vi "Rio_X_Motor_PID_Position_Control.vi"() -> ()   [LabVIEW 2017]
uses:
  <vilib>/myRIO/Common/Instrument Driver Framework/myRIO v1.0/Encoder/typedefs/Encoder Signal Mode.ctl
  <vilib>/myRIO/Instrument Drivers/Onboard IO/Encoder/typedefs/Encoder Reference.ctl
  <vilib>/myRIO/Common/Instrument Driver Framework/Utilities/typedefs/myRIO Generic Hardware Reference.ctl
  <vilib>/myRIO/Common/Instrument Driver Framework/Utilities/typedefs/Hardware Version Enum.ctl
  <vilib>/myRIO/Common/Instrument Driver Framework/Utilities/typedefs/myRIO v1.0 Reference.ctl
  <vilib>/myRIO/Common/Instrument Driver Framework/Utilities/typedefs/Generic FPGA Reference.ctl
  <vilib>/myRIO/Common/Instrument Driver Framework/myRIO v1.0/Encoder/typedefs/Encoder Channels Enum.ctl
  <vilib>/myRIO/Common/Instrument Driver Framework/myRIO v1.0/Encoder/typedefs/Encoder Configuration v1.0.ctl
  <vilib>/userdefined/High Color/nirio_resource_hc.ctl
  <vilib>/myRIO/Instrument Drivers/Onboard IO/DIO/typedefs/DIO Reference.ctl
  <vilib>/myRIO/Common/Instrument Driver Framework/myRIO v1.0/DIO/typedefs/DIO Channels List.ctl
  <vilib>/myRIO/Common/Instrument Driver Framework/myRIO v1.0/DIO/typedefs/DIO Channels Enum.ctl
  <vilib>/myRIO/Instrument Drivers/Onboard IO/PWM/typedefs/PWM Reference.ctl
  <vilib>/myRIO/Common/Instrument Driver Framework/myRIO v1.0/PWM/typedefs/PWM Channels Enum.ctl
  <vilib>/myRIO/Instrument Drivers/Onboard IO/PWM/typedefs/PWM Configuration.ctl
  <vilib>/myRIO/Common/Instrument Driver Framework/Utilities/vis/Is FPGA Ref Available.vi
  <vilib>/myRIO/Common/Instrument Driver Framework/myRIO v1.0/Encoder/vis/myRIO v1.1 Open Encoder.vi
  <vilib>/myRIO/Instrument Drivers/Onboard IO/Encoder/vis/Read.vi
  <vilib>/myRIO/Common/Instrument Driver Framework/myRIO v1.0/DIO/vis/myRIO v1.1 Open DIO.vi
  <vilib>/myRIO/Instrument Drivers/Onboard IO/DIO/vis/Write.vi
  <vilib>/myRIO/Common/Instrument Driver Framework/myRIO v1.0/PWM/vis/myRIO v1.1 Open PWM.vi
  <vilib>/myRIO/Instrument Drivers/Onboard IO/PWM/vis/Set Duty Cycle and Frequency.vi
  <vilib>/myRIO/Common/Instrument Driver Framework/Utilities/vis/Validate Channels.vi
  <vilib>/myRIO/Common/Instrument Driver Framework/myRIO v1.0/Encoder/vis/myRIO v1.0 Reserve Encoder.vi
  <vilib>/myRIO/Common/Instrument Driver Framework/myRIO v1.0/DIO/vis/myRIO v1.0 Reserve DIO.vi
  <vilib>/myRIO/Common/Instrument Driver Framework/myRIO v1.0/PWM/vis/myRIO v1.0 Reserve PWM.vi
  <vilib>/myRIO/Common/Instrument Driver Framework/myRIO v1.0/Encoder/vis/myRIO v1.0 Build MUX Configuration Encoder.vi
  <vilib>/myRIO/Common/Instrument Driver Framework/myRIO v1.0/Resource Manager/vis/myRIO v1.0 Reserve Channel List.vi
  <vilib>/myRIO/Common/Instrument Driver Framework/myRIO v1.0/DIO/vis/myRIO v1.0 Build MUX Configuration DIO.vi
  <vilib>/myRIO/Common/Instrument Driver Framework/myRIO v1.0/PWM/vis/myRIO v1.0 Build MUX Configuration PWM.vi
  <vilib>/myRIO/Common/Instrument Driver Framework/myRIO v1.0/Resource Manager/vis/myRIO v1.0 Create Configuration List.vi
  <vilib>/myRIO/Common/Instrument Driver Framework/myRIO v1.0/Resource Manager/vis/myRIO v1.0 Reserve Channel.vi
  <vilib>/myRIO/Common/Instrument Driver Framework/myRIO v1.0/Resource Manager/vis/myRIO v1.0 Unreserve Channel.vi
  <vilib>/myRIO/Common/Instrument Driver Framework/myRIO v1.0/Resource Manager/vis/myRIO v1.0 Build Mutex Name.vi
  <vilib>/Utility/VariantDataType/GetNumericInfo.vi
  <vilib>/Utility/error.llb/Error Cluster From Error Code.vi
  <vilib>/myRIO/Common/Instrument Driver Framework/myRIO v1.0/myRIO v1.1 Open.vi
  <vilib>/myRIO/Common/Instrument Driver Framework/Utilities/vis/IO Manager.vi
  <vilib>/myRIO/Common/Instrument Driver Framework/Utilities/vis/Configuration Manager.vi
  <vilib>/myRIO/Common/Instrument Driver Framework/myRIO v1.0/Resource Manager/vis/myRIO v1.0 Configure IO.vi
  <vilib>/myRIO/Common/Instrument Driver Framework/myRIO v1.0/myRIO v1.0 Close.vi
  <vilib>/myRIO/Common/Instrument Driver Framework/myRIO v1.0/Encoder/vis/myRIO v1.0 Configure Encoder.vi
  <vilib>/myRIO/Common/Instrument Driver Framework/myRIO v1.0/Encoder/vis/myRIO v1.0 Read Encoder.vi
  <vilib>/addons/control/pid/pid.llb/PID (DBL).vi
  <vilib>/myRIO/Common/Instrument Driver Framework/myRIO v1.0/DIO/vis/myRIO v1.0 Write DIO.vi
  <vilib>/myRIO/Common/Instrument Driver Framework/myRIO v1.0/PWM/vis/myRIO v1.0 Write PWM.vi
  <vilib>/myRIO/Express VI/Onboard IO/Encoder/Encoder Express VI.xnode
  <vilib>/myRIO/Instrument Drivers/Onboard IO/Encoder/vis/myRIO Encoder Open.xnode
  <vilib>/myRIO/Common/Instrument Driver Framework/myRIO v1.0/Encoder/typedefs/Encoder Count Direction Enum.ctl
  <vilib>/myRIO/Express VI/Onboard IO/DO/DO Express VI.xnode
  <vilib>/myRIO/Instrument Drivers/Onboard IO/DIO/vis/myRIO DIO Open.xnode
  <vilib>/myRIO/Express VI/Onboard IO/PWM/PWM Express VI.xnode
  <vilib>/myRIO/Instrument Drivers/Onboard IO/PWM/vis/myRIO PWM Open.xnode
  <vilib>/myRIO/Instrument Drivers/Onboard IO/Encoder/Encoder.lvlib
  <vilib>/addons/control/pid/NI_PID_pid.lvlib
  <vilib>/myRIO/Instrument Drivers/Onboard IO/PWM/PWM.lvlib
  <vilib>/myRIO/Instrument Drivers/Onboard IO/DIO/DIO.lvlib
  <vilib>/addons/control/pid/pid.llb/PID Control Input Filter (DBL).vi
panel:
  out "Waveform Chart":dbl[][](graph)
  in  "PID gains":T1={"proportional gain (Kc)"=1.0, "integral time (Ti, min)"=0.01, "derivative time (Td, min)"=0.0} {"derivative time (Td, min)" format="%.3f"; "integral time (Ti, min)" format="%.3f"; "proportional gain (Kc)" format="%.3f"}
  in  "setpoint":dbl format="%.2f"
  out "Counter Value 2":i32
  in  "stop 3":bool
  in  "stop 2":bool
  out "Error Out":errorcluster
  in  "Error In":errorcluster
  out "Waveform Graph":dbl[](graph)
  out "RPM Chart 2":cluster{"setpoint":dbl, dbl, "output":dbl}(graph)
  in  "Boolean":bool
  out "Time":dbl
  out "element":dbl
  in  "Controls":T2={"Start Pos"=0.0, "End Pos"=0.0, "Max V R/m"=100, "Accel Time (S)"=0.0}
  in  "stop":bool
  out "RPM Chart":dbl(graph)
  out "Counter Value":i32
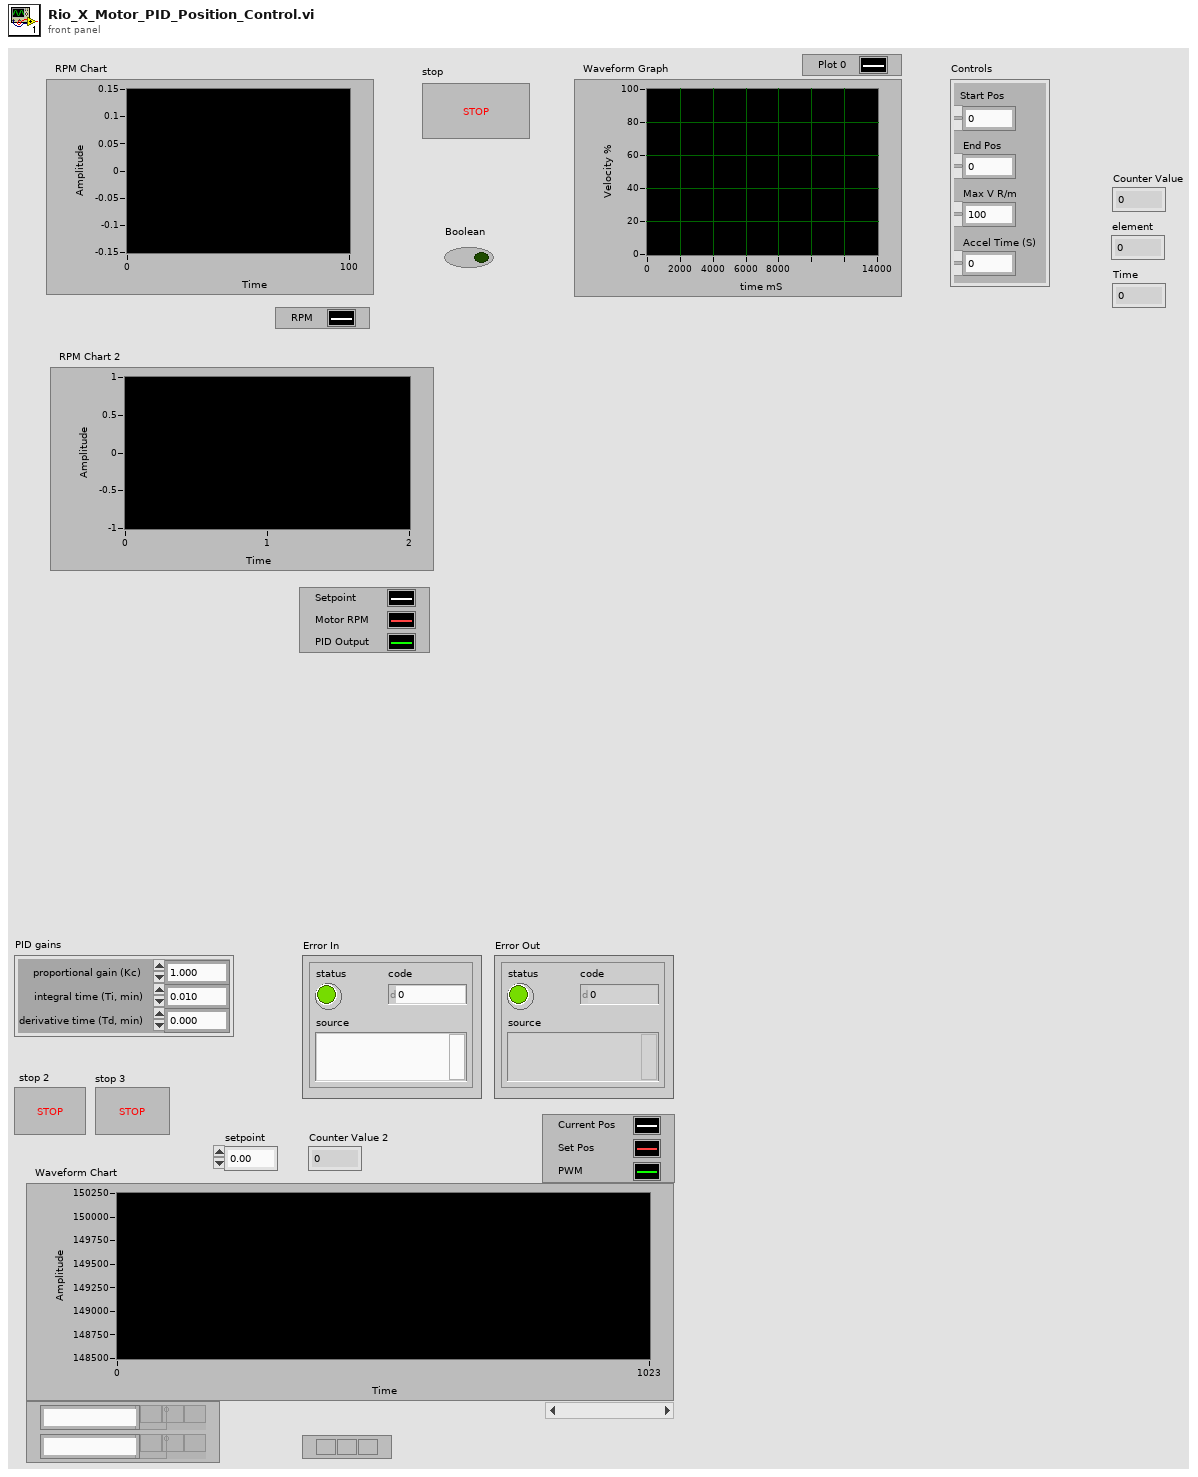
[diagram p1: front panel]
types:
  T1 = cluster{"proportional gain (Kc)":dbl, "integral time (Ti, min)":dbl, "derivative time (Td, min)":dbl}
  T2 = cluster{"Start Pos":dbl, "End Pos":dbl, "Max V R/m":i32, "Accel Time (S)":dbl}
  T3 = cluster{"X(t)/Y(f) Selection ":bool, "Duty Cycle (0-1) (X Control)":dbl, "Frequency [Hz] (Y Control)":dbl, "Direction (t:+, f:-)":bool}
  T4 = typedef "Encoder.lvlib/Encoder Reference.ctl" = cluster{"myRIO Reference":T5, "Encoder Channels Enum":T9}
  T5 = typedef "myRIO Generic Hardware Reference.ctl" = cluster{"myRIO Model":T6, "myRIO Hardware Reference":T7}
  T6 = typedef "Hardware Version Enum.ctl" = enum16{"Unknown", "myRIO-1900", "myRIO-1950", "roboRIO", "NI ELVIS RIO CM"}
  T7 = typedef "myRIO v1.0 Reference.ctl" = cluster{"Generic FPGA Reference":T8, "Allow multiple opens":bool}
  T8 = typedef "Generic FPGA Reference.ctl" = refnum<k20>
  T9 = typedef "Encoder Channels Enum.ctl" = enum16{"Not Connected", "C/ENC0", "C/ENC1", "A/ENC", "B/ENC", "DIO/ENC0", "DIO/ENC1", "DIO/ENC2", "DIO/ENC3", "DIO/ENC4"}
  T10 = typedef "Encoder Signal Mode.ctl" = enum16{"Quadrature phase signal", "Step and direction signal"}
  T11 = typedef "nirio_resource_hc.ctl" = tag
  T12 = cluster{"Boolean":bool, dbl, dbl, "Boolean":bool}
  T13 = typedef "DIO.lvlib/DIO Reference.ctl" = cluster{"myRIO Reference":T5, "DIO Channels List":T14}
  T14 = typedef "DIO Channels List.ctl" = T15[]
  T15 = typedef "DIO Channels Enum.ctl" = enum16{"Not Connected", "C/DIO0", "C/DIO1", "C/DIO2", "C/DIO3", "C/DIO4", "C/DIO5", "C/DIO6", "C/DIO7", "A/DIO0", "A/DIO1", "A/DIO2", "A/DIO3", "A/DIO4", "A/DIO5", "A/DIO6", "A/DIO7", "A/DIO8", "A/DIO9", "A/DIO10", "A/DIO11", "A/DIO12", "A/DIO13", "A/DIO14", "A/DIO15", "B/DIO0", "B/DIO1", "B/DIO2", "B/DIO3", "B/DIO4", "B/DIO5", "B/DIO6", "B/DIO7", "B/DIO8", "B/DIO9", "B/DIO10", "B/DIO11", "B/DIO12", "B/DIO13", "B/DIO14", "B/DIO15", "LED0", "LED1", "LED2", "LED3", "Button0", "DIO/DIO0", "DIO/DIO1", "DIO/DIO2", "DIO/DIO3", "DIO/DIO4", "DIO/DIO5", "DIO/DIO6", "DIO/DIO7", "DIO/DIO8", "DIO/DIO9", "SPI/CS0", "SPI/CS1", "SPI/CS2", "SPI/CS3", "LED RADIO (Green)", "LED RADIO (Red)", "LED COMM (Green)", "LED COMM (Red)", "LED MODE (Green)", "LED MODE (Red)"}
  T16 = typedef "PWM.lvlib/PWM Reference.ctl" = cluster{"myRIO Reference":T5, "PWM Channels Enum":T17, "PWM Configuration":T18}
  T17 = typedef "PWM Channels Enum.ctl" = enum16{"Not Connected", "C/PWM0", "C/PWM1", "A/PWM0", "A/PWM1", "A/PWM2", "B/PWM0", "B/PWM1", "B/PWM2", "PWM/PWM0", "PWM/PWM1", "PWM/PWM2", "PWM/PWM3", "PWM/PWM4", "PWM/PWM5", "PWM/PWM6", "PWM/PWM7", "PWM/PWM8", "PWM/PWM9"}
  T18 = typedef "PWM.lvlib/PWM Configuration.ctl" = cluster{"Frequency":dbl, "Duty Cycle":dbl}
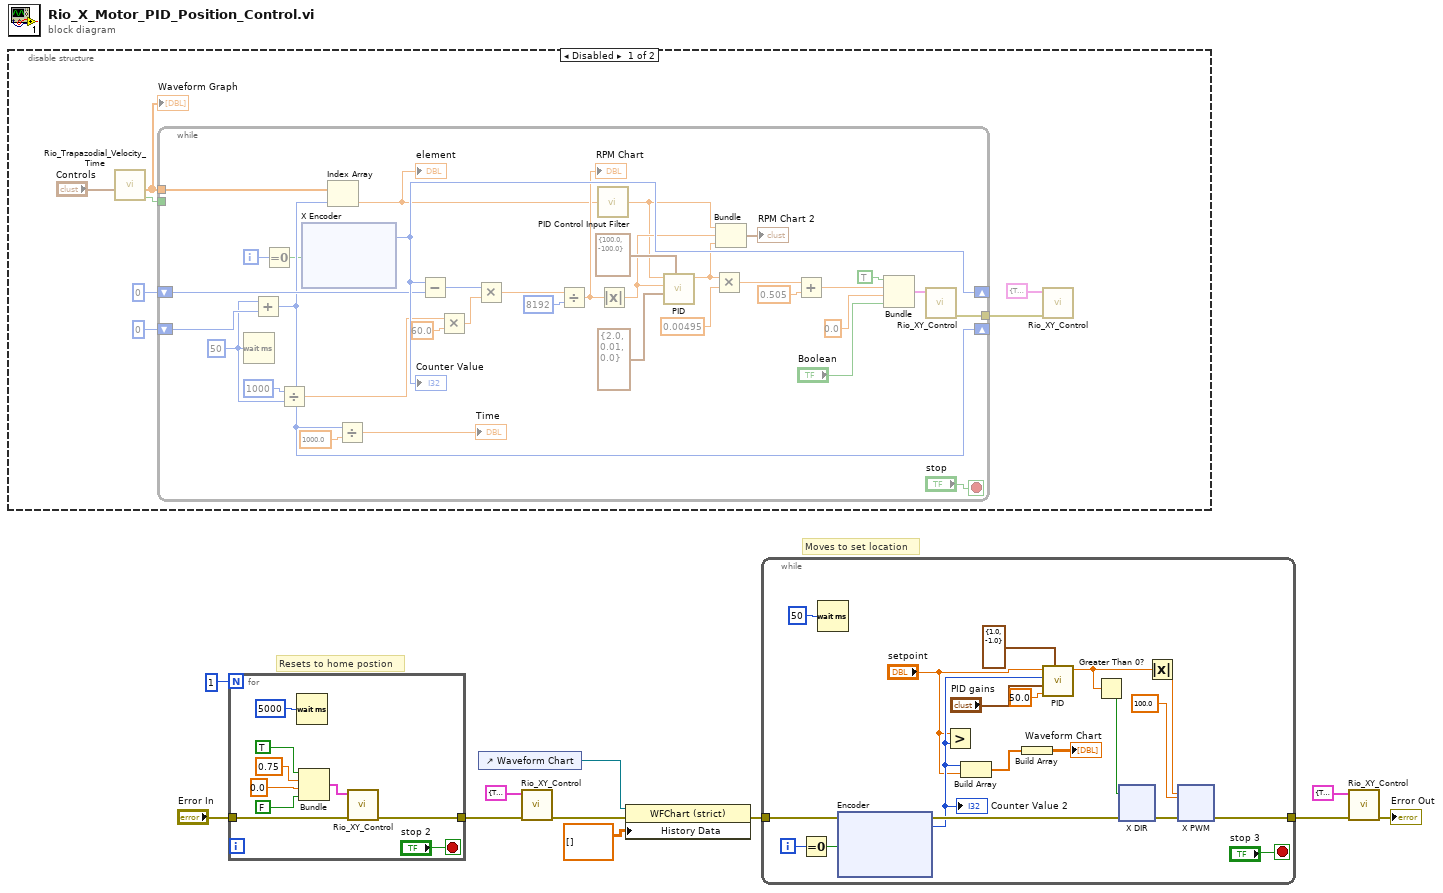
[diagram p0: block diagram]
diagram:
  # "Moves to set location"
  # "Resets to home postion"
  n1 = disable-structure shown="Disabled" {
    frame Disabled {
      n2 = call "Rio_Trapazodial_Velocity_Time.vi"("Controls"="Controls") -> ("Forward (t)/Reverse (f)"=w17:bool, "Waveform Graph"=w12:dbl[])  [unwired: 8 in, 1 out]
      "Waveform Graph" <- w12
      n3 = while {
        shift-right: [w49] -> _
        shift-left: 0 ("Counter Value") -> [w48]
        tunnel: w12 -> [w46]
        tunnel: w17 -> [_]
        shift-right: [w42] -> _
        shift-left: 0 -> [w45]
        tunnel: [w27] -> w15
        i -> [w25]
        stop <- "stop" stop-if-true
        w38 = u32 50 ("milliseconds to wait")
        n4 = Wait (ms)(milliseconds to wait=w38) -> ()  [unwired: 1 out]
        n5 = Add(x=w38, y=w45) -> (x+y=w42:u32)
        n6 = Equal To 0?(x=w25) -> (x = 0?=w20:bool)
        n7 = Divide(x=u32 1000, y=w38) -> (x/y=w44:dbl)
        n8 = xnode "X Encoder"("Reset Counter"=w20) -> ("Counter Value"=w49:i32)  [unwired: 1 in, 3 out]
        "Counter Value" <- w49
        n9 = Index Array(array=w46, index=w42) -> (element=w24:dbl)
        "element" <- w24
        n10 = Divide(x=w42, y=1000.0) -> (x/y=→"Time":dbl)
        n11 = Subtract(x=w49, y=w48) -> (x-y=w52:i32)
        n12 = Multiply(x=w44, y=60.0) -> (x*y=w39:dbl)
        n13 = Multiply(x=w52, y=w39) -> (x*y=w53:dbl)
        n14 = Divide(x=w53, y=8192) -> (x/y=w26:dbl)
        "RPM Chart" <- w26
        n15 = call-poly <vilib>:"PID Control Input Filter.vi"("input"=w24) -> ("output"=w19:dbl)  [unwired: 4 in]
        n16 = Absolute Value(x=w26) -> (abs(x)=w23:dbl)
        n17 = call-poly <vilib>:"PID.vi"("output range"=cluster{"output high":dbl, "output low":dbl} {"output high"=100.0, "output low"=-100.0}, "PID gains"=T1 {"proportional gain (Kc)"=2.0, "integral time (Ti, min)"=0.01, "derivative time (Td, min)"=0.0}, "process variable"=w23, "setpoint"=w19) -> ("output"=w22:dbl)  [unwired: 6 in, 1 out]
        n18 = Multiply(x=w22, y=0.00495) -> (x*y=w35:dbl)
        n19 = Bundle("output"=w19, w23, "output"=w22) -> (→"RPM Chart 2":cluster{"output":dbl, dbl, "output":dbl})  [unwired: 1 in]
        n20 = Add(x=w35, y=0.505) -> (x+y=w29:dbl)
        n21 = Bundle("Boolean"=TRUE, w29, 0.0, "Boolean"="Boolean") -> (w30:T12)  [unwired: 1 in]
        n22 = call "Rio_XY_Control.vi"("Input Cluster"=w30) -> ("Error Out"=w27:errorcluster)  [unwired: 10 in]
      }
      n23 = call "Rio_XY_Control.vi"("Error In"=w15, "Input Cluster"=T3 {"X(t)/Y(f) Selection "=TRUE, "Duty Cycle (0-1) (X Control)"=0.0, "Frequency [Hz] (Y Control)"=0.0, "Direction (t:+, f:-)"=TRUE}) -> ()  [unwired: 9 in, 1 out]
    }
    frame Enabled {
    }
  }
  n24 = for {
    N: 1 -> [_]
    tunnel: "Error In" -> [w102]
    tunnel: [w101] -> w9
    stop <- "stop 2" stop-if-true
    n25 = Wait (ms)(milliseconds to wait=u32 5000) -> ()  [unwired: 1 out]
    n26 = Bundle("Boolean"=TRUE, 0.75, 0.0, "Boolean"=FALSE) -> (w106:T12)  [unwired: 1 in]
    n27 = call "Rio_XY_Control.vi"("Error In"=w102, "Input Cluster"=w106) -> ("Error Out"=w101:errorcluster)  [unwired: 9 in]
  }
  n28 = control-ref of="Waveform Chart"() -> (w3:refnum<vi>)
  n29 = call "Rio_XY_Control.vi"("Error In"=w9, "Input Cluster"=T3 {"X(t)/Y(f) Selection "=TRUE, "Duty Cycle (0-1) (X Control)"=0.0, "Frequency [Hz] (Y Control)"=0.0, "Direction (t:+, f:-)"=TRUE}) -> ("Error Out"=w2:errorcluster)  [unwired: 9 in]
  n30 = property class="WFChart (strict)"(reference=w3, error in=w2, "History Data"=dbl[][] []) -> (error out=w1:errorcluster)  [unwired: 1 out]
  n31 = while {
    tunnel: w1 -> [w126]
    tunnel: [w124] -> w5
    i -> [w119]
    stop <- "stop 3" stop-if-true
    n32 = Equal To 0?(x=w119) -> (x = 0?=w117:bool)
    n33 = Wait (ms)(milliseconds to wait=u32 50) -> ()  [unwired: 1 out]
    n34 = xnode "Encoder"("error in (no error)"=w126, "Reset Counter"=w117) -> ("error out"=w125:errorcluster, "Counter Value"=w121:i32)  [unwired: 2 out]
    "Counter Value 2" <- w121
    n35 = Greater?(x="setpoint", y=w121) -> ()  [unwired: 1 out]
    n36 = Build Array(w121, "setpoint") -> (w123:dbl[])
    n37 = Build Array(w123) -> (→"Waveform Chart":dbl[][])
    n38 = call-poly <vilib>:"PID.vi"("output range"=cluster{"output high":dbl, "output low":dbl} {"output high"=1.0, "output low"=-1.0}, "dt (s)"=50.0, "PID gains"="PID gains", "process variable"=w121, "setpoint"="setpoint") -> ("output"=w111:dbl)  [unwired: 5 in, 1 out]
    n39 = Greater Than 0?(x=w111) -> (x > 0?=w110:bool)
    n40 = xnode "X DIR"("error in (no error)"=w125, "X Axis Direction (A/DIO4 (Pin 19))"=w110) -> ("error out"=w112:errorcluster)
    n41 = Absolute Value(x=w111) -> (abs(x)=w109:dbl)
    n42 = xnode "X PWM"("error in (no error)"=w112, "Duty Cycle"=w109, "Frequency [Hz]"=100.0) -> ("error out"=w124:errorcluster)
  }
  n43 = call "Rio_XY_Control.vi"("Error In"=w5, "Input Cluster"=T3 {"X(t)/Y(f) Selection "=TRUE, "Duty Cycle (0-1) (X Control)"=0.0, "Frequency [Hz] (Y Control)"=0.0, "Direction (t:+, f:-)"=TRUE}) -> ("Error Out"=→"Error Out":errorcluster)  [unwired: 9 in]
